vi "PWM Latched.vi"() -> ()   [LabVIEW 2015]
doc: "This VI uses a PWM Out Latched (subVI).vi to generate a pulse train on DIO 0 according to the Low Period and High Period controls. Changes in the Low Period (ms) and High Period (ms) controls take effect on the next full period following the assertion Load boolean.\n\nIt then uses PWM In (subVI).vi to measure DIO 1 and report the measured Low Period and High Period. The measurements indicate the first full period after the Latch button is asserted.\n\nHardware Connection Required - Use a wire to physically connect DIO0 to DIO1."
uses:
  <vilib>/Platform/TimedLoop/XDataNode/timing_clust.ctl
  <vilib>/Platform/TimedLoop/XDataNode/nitl_modes.ctl
  <vilib>/Platform/TimedLoop/XDataNode/wakeup.ctl
  <vilib>/rvi/Emulation/niFpgaGetClockAttributes.vi
  <vilib>/rvi/Emulation/niFpgaSctlEmulationGetInTimedLoop.vi
  <vilib>/rvi/Emulation/niFpgaEmulationReportErrorSimple.vi
  <vilib>/rvi/eio/common/nirviEmuTemplateMethod_errors.vi
  <vilib>/rvi/Emulation/niFpgaCriticalErrorInLSC.vi
  <vilib>/eio/EIONode/EIONode.xnode
  <vilib>/Platform/TimedLoop/XDataNode/XDataNode.xnode
  <vilib>/Platform/TimedLoop/XDataNode/XDNodeRunTimeDep.lvlib
panel:
  in  "Stop Input":bool
  out "LED Indicator":bool
  in  "Latch":bool
  out "Low Period (ms)":u32=500
  out "High Period (ms)":u32=500
  in  "Run":bool=TRUE
  in  "Load":bool
  in  "Low Period (ms)":u16=500
  in  "High Period (ms)":u16=500
  in  "Stop Output":bool
  # "This VI uses a PWM Out Latched (subVI).vi to generate a pulse train on DIO 0 according to the\nLow Period and High Period controls, when Run is true. Changes in the Low Period (ms) and \nHigh Period (ms) controls take effect on the next full period following pressing the Load control.\n\nIt then uses PWM In (subVI).vi to measure DIO 1 and report the measured Low Period and \nHigh Period.  The measurements are updated only after the Latch control is asserted.\n\nHardware Connection Required - Use a wire to physically connect DIO0 to DIO1."
  # "Output"
  # "Measure"
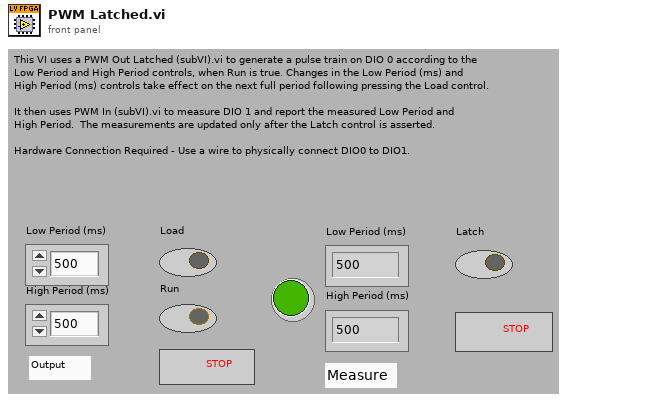
[diagram p1: front panel]
types:
  T1 = typedef "XDNodeRunTimeDep.lvlib/timing_clust.ctl" = cluster{"Expected End [f-1]":u64, "Actual End [f-1]":u64, "Finished Late? [f-1]":bool, "Expected End [i-1]":u64, "Actual End [i-1]":u64, "Finished Late? [i-1]":bool, "Expected Start [i]":u64, "Actual Start [i]":u64, "Expected Start [f]":u64, "Actual Start [f]":u64, "Source Name":string, "Structure Name":string, "Period":i64, "Deadline":i64, "Offset":i64, "Start":i64, "Priority":i32, "Timeout":i32, "Mode":T2, "Wakeup Reason":T3, "Error":errorcluster, "Source Type":string, "Secondary Source Type":string, "Global End Time":u64, "Global Start Time":u64, "Frame Duration":u64, "Iteration Duration":u64, "Assigned CPU":i32, "I/O Scan Engine Mode":u32}
  T2 = typedef "XDNodeRunTimeDep.lvlib/nitl_modes.ctl" = enum32{"No Change", "Process missed periods, maintain original phase", "Discard missed periods, maintain original phase", "Process missed periods, ignore original phase", "Discard missed periods, ignore original phase"}
  T3 = typedef "XDNodeRunTimeDep.lvlib/wakeup.ctl" = enum32{"Normal", "Aborted", "Asynchronous wakeup", "Timing source error", "Timed loop error", "Timeout"}
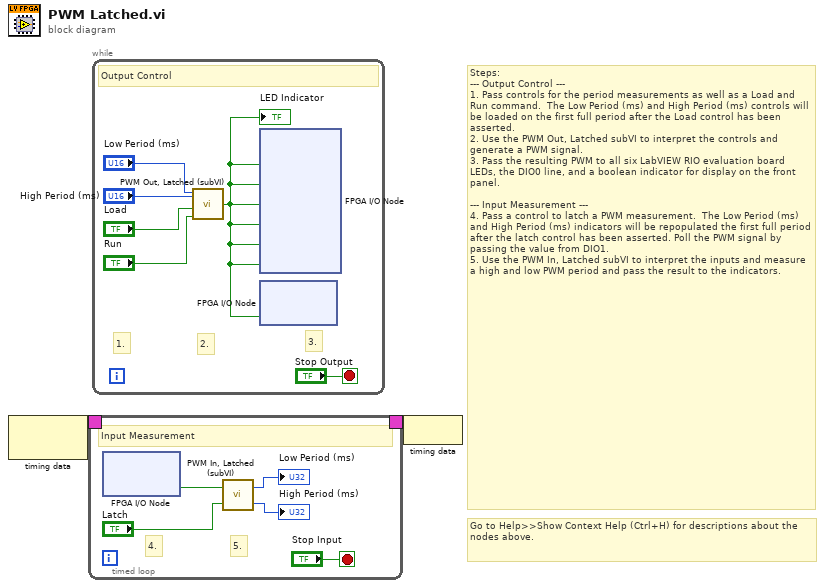
[diagram p0: block diagram]
diagram:
  # "Go to Help>>Show Context Help (Ctrl+H) for descriptions about the nodes above."
  # "Steps:\n--- Output Control ---\n1. Pass controls for the period measurements as well as a Load and Run command.  The Low Period (ms) and High Period (ms) controls will be loaded on the first full period after the Load control has been asserted.\n2. Use the PWM Out, Latched subVI to interpret the controls and generate a PWM signal.\n3. Pass the resulting PWM to all six LabVIEW RIO evaluation board LEDs, the DIO0 line, and a boolean indicator for display on the front panel. \n\n--- Input Measurement ---\n4. Pass a control to latch a PWM measurement.  The Low Period (ms) and High Period (ms) indicators will be repopulated the first full period after the latch control has been asserted. Poll the PWM signal by passing the value from DIO1.\n5. Use the PWM In, Latched subVI to interpret the inputs and measure a high and low PWM period and pass the result to the indicators."
  n1 = node-c288() -> (w2:T1)  [unwired: 1 out]
  n2 = timed-loop {
    timing: w2 -> [_]
    timing-out: [_] -> w1
    stop <- "Stop Input" stop-if-true
    # "5."
    # "4."
    # "Input Measurement"
    n3 = xnode "FPGA I/O Node"() -> ("DIO1"=w4:bool)  [unwired: 1 in, 1 out]
    n4 = call "PWM In, Latched (subVI).vi"("Latch"="Latch", "Input"=w4) -> ("High Period"=→"High Period (ms)":u32, "Low Period"=→"Low Period (ms)":u32)
  }
  n5 = while {
    stop <- "Stop Output" stop-if-true
    # "3."
    # "2."
    # "1."
    # "Output Control"
    n6 = call "PWM Out, Latched (subVI).vi"("Low Period"="Low Period (ms)", "High Period"="High Period (ms)", "Load"="Load", "Run"="Run") -> ("PWM Output"=w10:bool)  [unwired: 4 out]
    "LED Indicator" <- w10
    n7 = xnode "FPGA I/O Node"("LED 1"=w10, "LED 2"=w10, "LED 3"=w10, "LED 4"=w10, "LED 5"=w10, "LED 6"=w10) -> ()  [unwired: 6 in, 6 out]
    n8 = xnode "FPGA I/O Node"("DIO0"=w10) -> ()  [unwired: 1 in, 1 out]
  }
  n9 = node-c288(w1) -> ()
